vi "GetBlockTable.vi"(8 "Right Block":bool, 9 "Left Block":bool, 10 "Catch Index":dbl, 11 "Proc Index":dbl) -> (0 "Time":i32, 1 "B":i32, 2 "A":i32, 3 "CMD":i32)   [LabVIEW 2018]
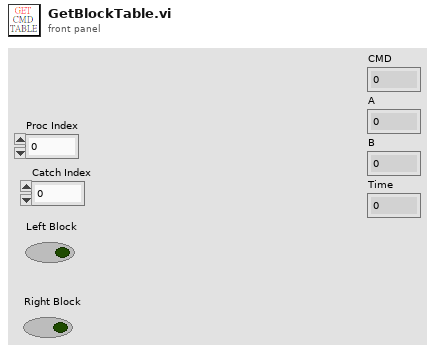
[diagram p1: front panel]
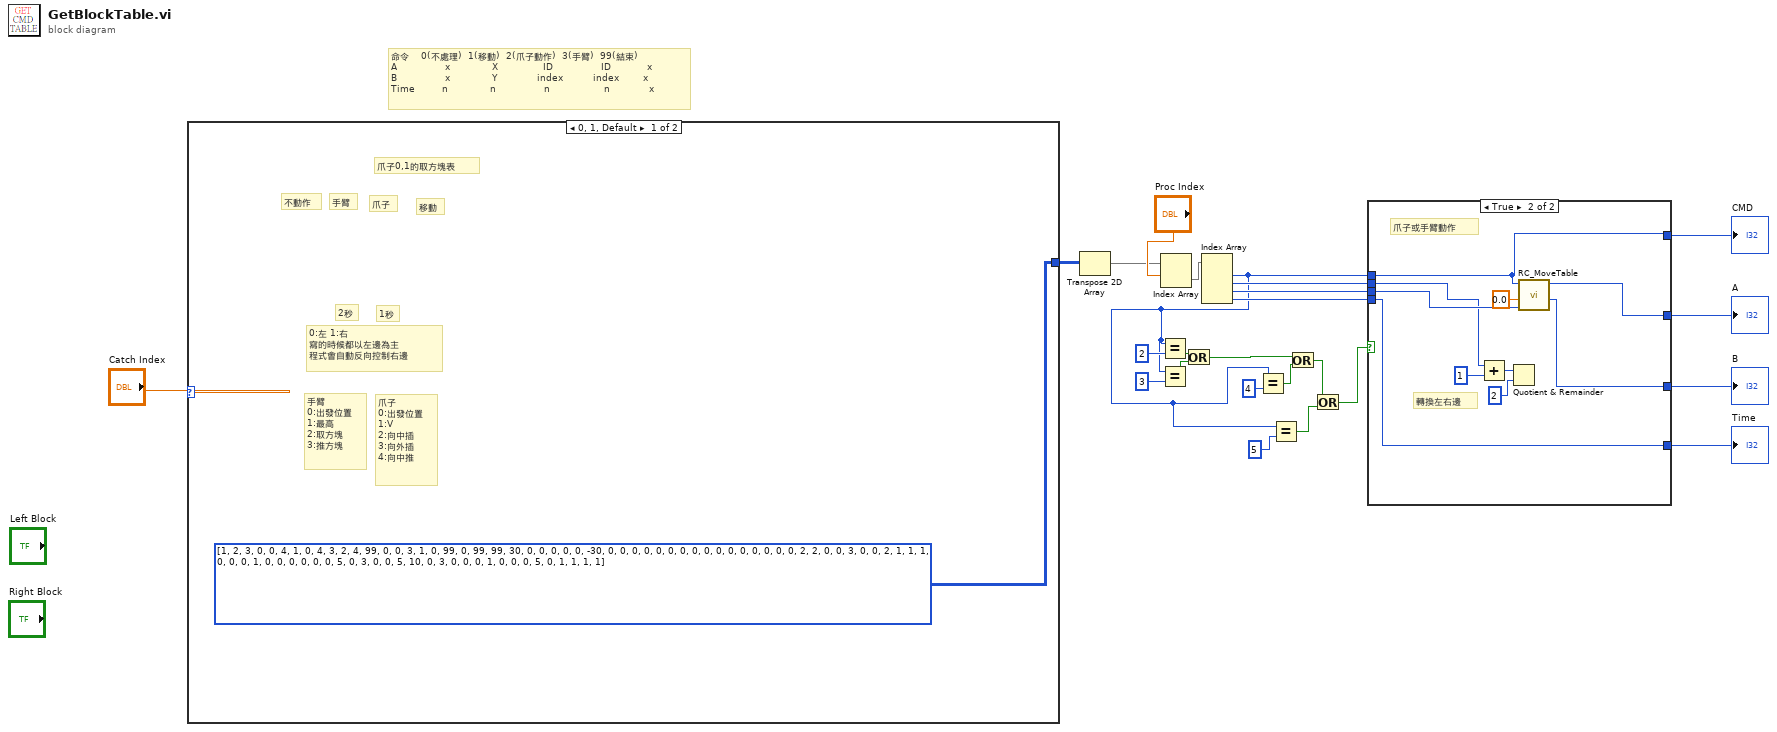
[diagram p0: block diagram]
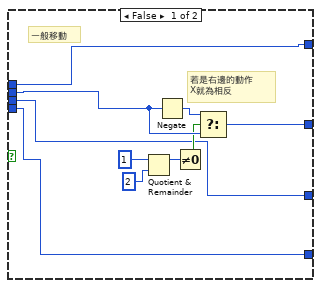
[diagram p2: hidden frame]
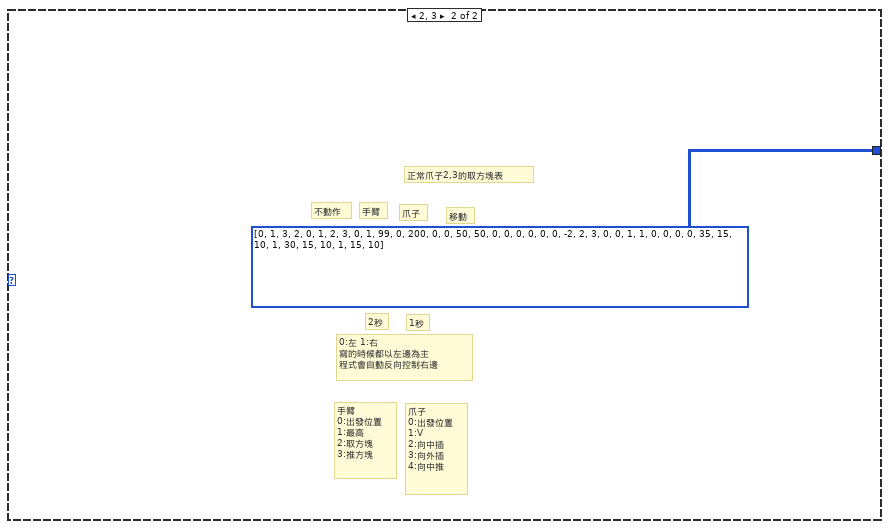
[diagram p3: hidden frame]
diagram:
  # "命令    0(不處理)  1(移動)  2(爪子動作)  3(手臂)  99(結束)\nA                x              X               ID                ID            x\nB                x              Y             index          index        x\nTime         n              n                n                  n             x"
  n1 = case shown="0, 1, Default" "Catch Index" {
    tunnel: [i32[][] [[1, 2, 3, 0, 0, 4, 1, 0, 4, 3, 2, 4, 99, 0, 0, 3, 1, 0, 99, 0, 99, 99], [30, 0, 0, 0, 0, 0, -30, 0, 0, 0, 0, 0, 0, 0, 0, 0, 0, 0, 0, 0, 0, 0], [0, 2, 2, 0, 0, 3, 0, 0, 2, 1, 1, 1, 0, 0, 0, 1, 0, 0, 0, 0, 0, 0], [5, 0, 3, 0, 0, 5, 10, 0, 3, 0, 0, 0, 1, 0, 0, 0, 5, 0, 1, 1, 1, 1]] i32[][] [[0, 1, 3, 2, 0, 1, 2, 3, 0, 1, 99], [0, 200, 0, 0, 50, 50, 0, 0, 0, 0, 0], [0, -2, 2, 3, 0, 0, 1, 1, 0, 0, 0], [0, 35, 15, 10, 1, 30, 15, 10, 1, 15, 10]]] -> w10
    frame 0, 1, Default {
      # "手臂\n0:出發位置\n1:最高\n2:取方塊\n3:推方塊"
      # "爪子\n0:出發位置\n1:V\n2:向中插\n3:向外插\n4:向中推"
      # "0:左 1:右 \n寫的時候都以左邊為主\n程式會自動反向控制右邊"
      # "爪子"
      # "移動"
      # "不動作"
      # "1秒"
      # "2秒"
      # "手臂"
      # "爪子0,1的取方塊表"
    }
    frame 2, 3 {
      # "手臂\n0:出發位置\n1:最高\n2:取方塊\n3:推方塊"
      # "爪子\n0:出發位置\n1:V\n2:向中插\n3:向外插\n4:向中推"
      # "0:左 1:右 \n寫的時候都以左邊為主\n程式會自動反向控制右邊"
      # "爪子"
      # "移動"
      # "不動作"
      # "1秒"
      # "2秒"
      # "手臂"
      # "正常爪子2,3的取方塊表"
    }
  }
  n2 = Transpose 2D Array(2D array=w10) -> (transposed array=w9:i32[][])
  n3 = Index Array(array=w9, index (row)="Proc Index") -> (element=w11:i32[])  [unwired: 1 in]
  n4 = Index Array(array=w11) -> (element #1=w5:i32, element #2=w22:i32, element #3=w21:i32, element #4=w20:i32)  [unwired: 4 in]
  n5 = Equal?(x=w5, y=2) -> (x = y?=w17:bool)
  n6 = Equal?(x=w5, y=3) -> (x = y?=w16:bool)
  n7 = Or(x=w17, y=w16) -> (x .or. y?=w8:bool)
  n8 = Equal?(x=w5, y=4) -> (x = y?=w7:bool)
  n9 = Equal?(x=w5, y=5) -> (x = y?=w3:bool)
  n10 = Or(x=w8, y=w7) -> (x .or. y?=w2:bool)
  n11 = Or(x=w2, y=w3) -> (x .or. y?=w1:bool)
  n12 = case shown="True" w1 {
    tunnel: w5 -> [w34 w39]
    tunnel: w22 -> [w32 w45]
    tunnel: w21 -> [w29 w46]
    tunnel: w20 -> [w28 w40]
    tunnel: [w34 w39] -> w15
    tunnel: [w30 w42] -> w14
    tunnel: [w29 w41] -> w13
    tunnel: [w28 w40] -> w12
    frame False {
      # "一般移動"
      # "若是右邊的動作\nX就為相反"
      n13 = Quotient & Remainder(x=1, y=2) -> (x-y*floor(x/y)=w35:i32)  [unwired: 1 out]
      n14 = Negate(x=w32) -> (-x=w33:i32)
      n15 = Not Equal To 0?(x=w35) -> (x != 0?=w31:bool)
      n16 = Select(t=w33, s=w31, f=w32) -> (s? t:f=w30:i32)
    }
    frame True {
      # "爪子或手臂動作"
      # "轉換左右邊"
      n17 = Add(x=w45, y=1) -> (x+y=w44:i16)
      n18 = Quotient & Remainder(x=w44, y=2) -> ()  [unwired: 2 out]
      n19 = call "RC_MoveTable.vi"("Index"=w46, "ID"=0.0, "CMD"=w39) -> ("Value"=w41:i32, "RC ID"=w42:i32)  [unwired: 6 in]
    }
  }
  "CMD" <- w15
  "A" <- w14
  "B" <- w13
  "Time" <- w12
